vi "Build Tree From Data (Recursive).vi"(8 "error in (no error)":errorcluster, 9 "Variant":variant, 10 "Parent Tag (empty)":string, 11 "TreeControl Ref":refnum<vi>) -> (0 "error out":errorcluster, 1 "Leaf-Level?":bool, 3 "TreeControl Ref":refnum<vi>)   [LabVIEW 2015]
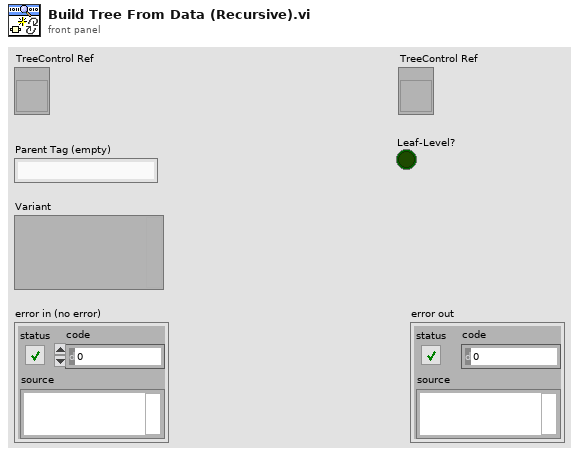
[diagram p1: front panel]
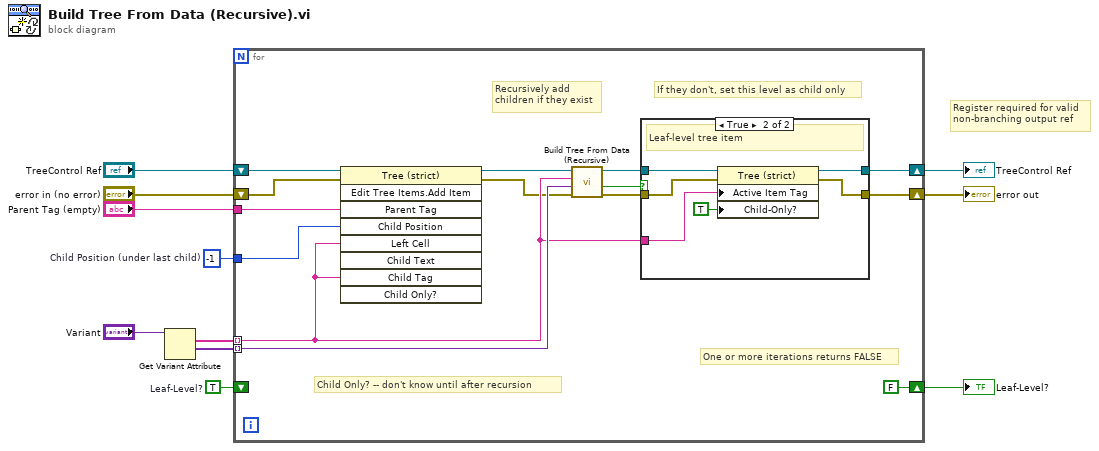
[diagram p0: block diagram]
diagram:
  w1 = TRUE  # Leaf-Level?
  w2 = -1  # Child Position (under last child)
  # "Register required for valid\nnon-branching output ref"
  n1 = Get Variant Attribute(Variant="Variant") -> (names=w4:string[], values=w3:variant[])  [unwired: 3 in, 2 out]
  n2 = for {
    tunnel: w3 -> [w22] mode=indexing
    shift-right: [w21] -> w10
    shift-left: "error in (no error)" -> [w25]
    tunnel: "Parent Tag (empty)" -> [w24]
    tunnel: w4 -> [w19] mode=indexing
    shift-right: [w20] -> w6
    shift-left: "TreeControl Ref" -> [w12]
    tunnel: w2 -> [w23]
    shift-right: [FALSE ("Leaf-Level?")] -> w5
    shift-left: w1 -> [_]
    # "Child Only? -- don't know until after recursion"
    # "If they don't, set this level as child only"
    # "One or more iterations returns FALSE"
    # "Recursively add\nchildren if they exist"
    n3 = invoke class="Tree (strict)" method="Edit Tree Items.Add Item"(reference=w12, error in=w25, "Parent Tag"=w24, "Child Position"=w23, "Left Cell"=w19, "Child Tag"=w19) -> (reference out=w16:refnum<vi>, error out=w17:errorcluster)  [unwired: 3 in, 7 out]
    n4 = call "Build Tree From Data (Recursive).vi"("error in (no error)"=w17, "Variant"=w22, "Parent Tag (empty)"=w19, "TreeControl Ref"=w16) -> ("error out"=w13:errorcluster, "Leaf-Level?"=w15:bool, "TreeControl Ref"=w14:refnum<vi>)  [unwired: 5 in]
    n5 = case shown="True" w15 {
      tunnel: w14 -> [w27 w33]
      tunnel: w13 -> [w26 w32]
      tunnel: [w26 w31] -> w21
      tunnel: [w27 w30] -> w20
      tunnel: w19 -> [_ w28]
      frame False {
        # "Not leaf-level (skip prop node call)"
      }
      frame True {
        # "Leaf-level tree item"
        n6 = property class="Tree (strict)"(reference=w33, error in=w32, "Active Item Tag"=w28, "Child-Only?"=TRUE ("Active Item:Child-Only?")) -> (reference out=w30:refnum<vi>, error out=w31:errorcluster)
      }
    }
  }
  "error out" <- w10
  "TreeControl Ref" <- w6
  "Leaf-Level?" <- w5
